vi "rqcAlice Modulator DAC Configure.vi"(8 "error in":errorcluster, 10 "RndGen.parameters":T1={"value type"=enum."constant", "constant"=0, "num of levels"=0, "levels values"=[0, 0, 0, 0]} {"num of levels" min=4 max=4 step=1}, 11 "Alice FPGA Reference In":refnum<k20>) -> (0 "error out":errorcluster, 3 "Alice FPGA Reference Out":refnum<k20>)   [LabVIEW 2019]
uses:
  Shared/Shared FPGA Lib/Shared Logic/Custom Controls/rqc Random Generator.parameters.ctl
  Shared/Shared FPGA Lib/Shared Logic/Custom Controls/rqc Random Generator.value type.ctl
  <vilib>/Utility/error.llb/Error Cluster From Error Code.vi
  <vilib>/rvi/errors/niLvFpgaAdjustHostInterfaceError.vi
  <vilib>/rvi/interface/nirviReadWriteControl/nirviReadWriteControl.xnode
  NiFpgaLv.dll
  <vilib>/rvi/interface/Simulation/niFpgaSimulationCallBeginRW.vi
panel:
  # "Constant"
  # "Random"
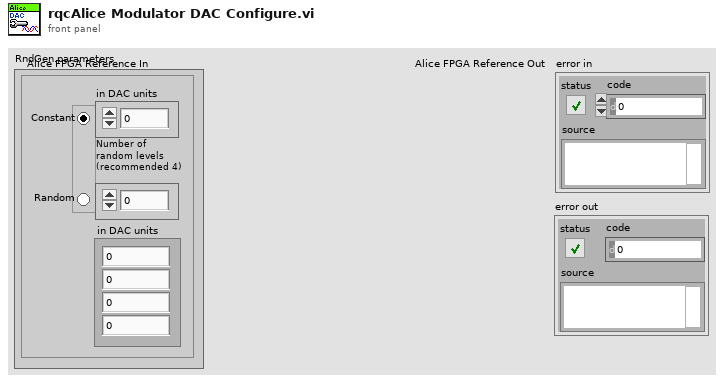
[diagram p1: front panel]
types:
  T1 = typedef "rqc Random Generator.parameters.ctl" = cluster{"value type":T2, "constant":u16, "num of levels":u16, "levels values":u16[]}
  T2 = typedef "rqc Random Generator.value type.ctl" = enum32{"random value", "constant"}
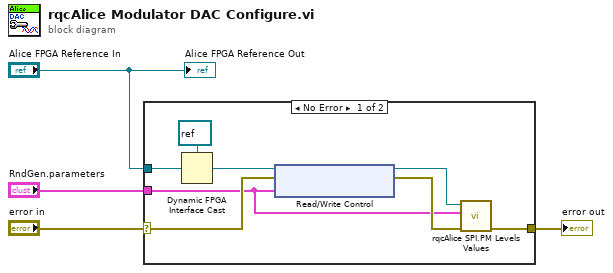
[diagram p0: block diagram]
diagram:
  n1 = case shown="No Error" "error in" {
    selector: "error in" -> [w9 w13]
    tunnel: [w5 w13] -> w3
    tunnel: "Alice FPGA Reference In" -> [w12 _]
    tunnel: "RndGen.parameters" -> [w7 _]
    frame No Error {
      n2 = Dynamic FPGA Interface Cast(Session In=refnum<k20> refnum ("Type"), Type=w12) -> (Session Out=w10:refnum<k20>)
      n3 = xnode "Read/Write Control"("FPGA VI Reference In"=w10, "error in"=w9, "rndGen.parameters"=w7) -> ("FPGA VI Reference Out"=w6:refnum<k20>, "error out"=w8:errorcluster)
      n4 = call "rqcAlice SPI.PM Levels Values.vi"("error in"=w8, "RndGen.parameters"=w7, "Alice FPGA Reference In"=w6) -> ("error out"=w5:errorcluster)  [unwired: 6 in, 2 out]
    }
    frame Error {
    }
  }
  "error out" <- w3
  "Alice FPGA Reference Out" <- "Alice FPGA Reference In"
